vi "Digitizer_Mode_Read.vi"(8 "error in":errorcluster, 11 "Channel Parameters In":T1) -> (0 "error out":errorcluster, 1 "Waveforms Out":T2(array[cluster]), 2 "Ch1_Plot":dbl[](array[numeric]), 3 "dup Channel Parameters Out":T1)   [LabVIEW 2010]
uses:
  Typedef-Channel Parameters.ctl
  <instrlib>/niScope/Acquire/Fetch/niScope Multi Fetch Cluster.vi
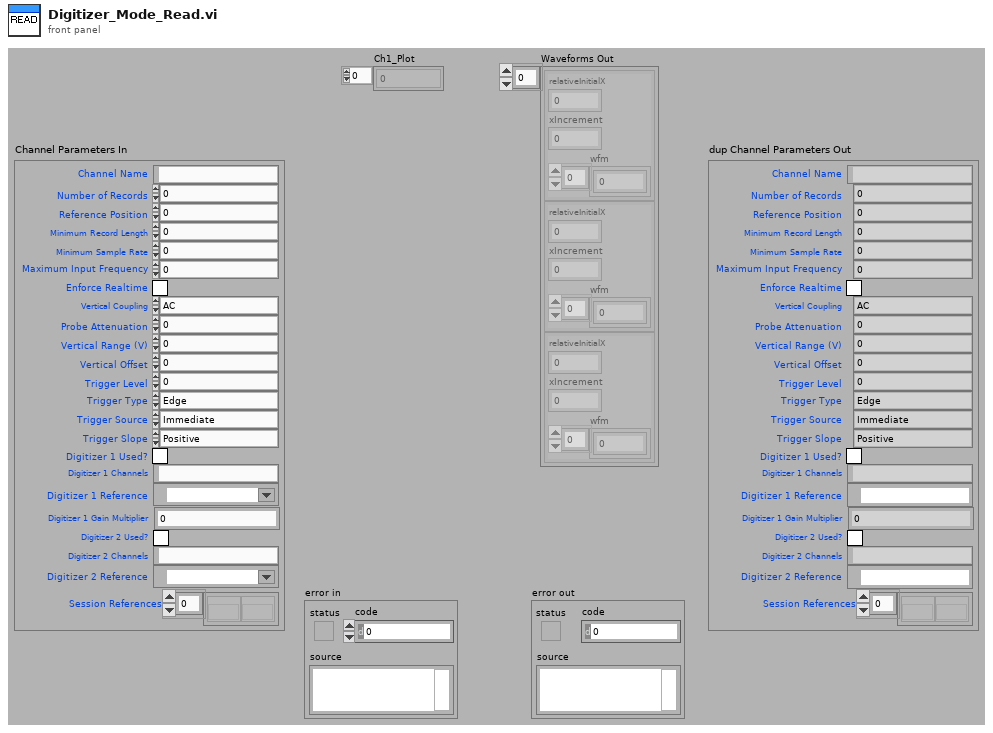
[diagram p1: front panel]
types:
  T1 = typedef "Typedef-Channel Parameters.ctl" = cluster{"Channel Name":string, "Number of Records":i32, "Reference Position":dbl, "Minimum Record Length":i32, "Minimum Sample Rate":dbl, "Maximum Input Frequency":dbl, "Enforce Realtime":bool, "Vertical Coupling":enum16{"AC", "DC", "Ground"}, "Probe Attenuation":dbl, "Vertical Range (V)":dbl, "Vertical Offset":dbl, "Trigger Level":dbl, "Trigger Type":enum16{"Edge", "Digital", "Immediate"}, "Trigger Source":enum16{"Immediate", "Channel 0", "Channel 1", "Channel 2", "Channel 3", "Channel 4", "Channel 5", "Channel 6", "Channel 7", "Extermal TRIG", "Software Trigger", "RTSI 0", "RTSI 1", "RTSI 2", "RTSI 3", "RTSI 4", "RTSI 5", "RTSI 6", "PF 0", "PF 1", "PF 2", "PXI Star Trigger"}, "Trigger Slope":enum16{"Positive", "Negative"}, "Digitizer 1 Used?":bool, "Digitizer 1 Channels":string, "Digitizer 1 Reference":refnum<k15>, "Digitizer 1 Gain Multiplier":dbl, "Digitizer 2 Used?":bool, "Digitizer 2 Channels":string, "Digitizer 2 Reference":refnum<k15>, "Session References":refnum<k20>[]}
  T2 = cluster{"relativeInitialX":dbl, "xIncrement":dbl, "wfm":dbl[]}[]
  T3 = cluster{"relativeInitialX":dbl, "xIncrement":dbl, "wfm":dbl[]}
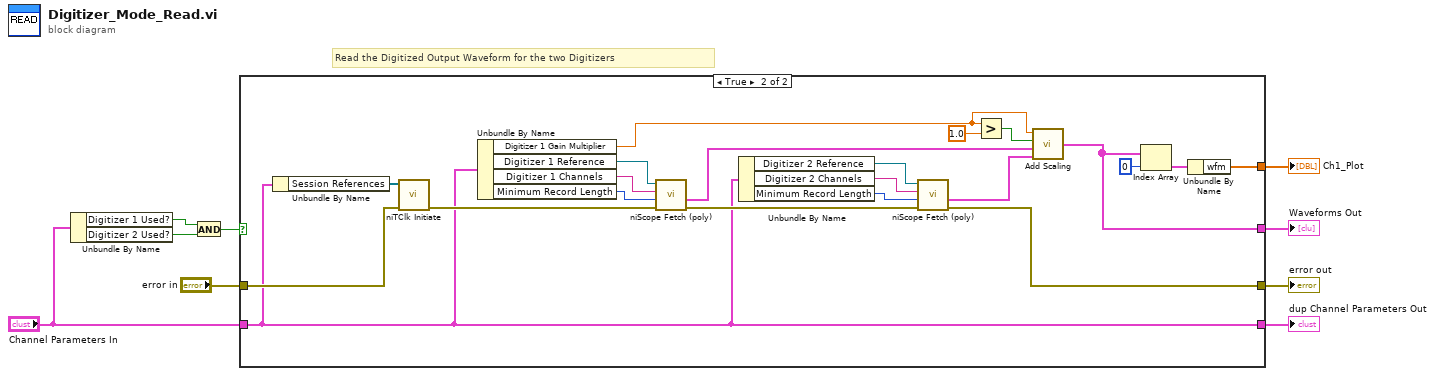
[diagram p0: block diagram]
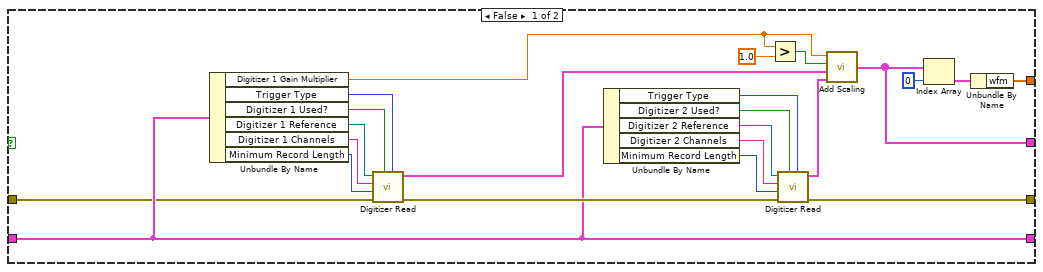
[diagram p2: hidden frame]
diagram:
  # "Read the Digitized Output Waveform for the two Digitizers"
  n1 = Unbundle By Name("Channel Parameters In") -> ("Digitizer 1 Used?"=w6:bool, "Digitizer 2 Used?"=w5:bool)
  n2 = And(x=w6, y=w5) -> (x .and. y?=w3:bool)
  n3 = case shown="True" w3 {
    tunnel: [w30 w35] -> w9
    tunnel: [w27 w39] -> w8
    tunnel: [w16 w36] -> w7
    tunnel: "Channel Parameters In" -> [w11 w33]
    tunnel: [w11 w33] -> w2
    tunnel: "error in" -> [w10 w53]
    frame False {
      n4 = Unbundle By Name(w11) -> ("Digitizer 1 Gain Multiplier"=w32:dbl, "Trigger Type"=w17:enum16{"Edge", "Digital", "Immediate"}, "Digitizer 1 Used?"=w18:bool, "Digitizer 1 Reference"=w13:refnum<k15>, "Digitizer 1 Channels"=w19:string, "Minimum Record Length"=w20:i32)
      n5 = call "Digitizer Read.vi"("Trigger Type"=w17, "Dig Used"=w18, "error in"=w10, "Min Record Length"=w20, "Dig Channels"=w19, "Dig Ref"=w13) -> ("error out"=w21:errorcluster, "waveform out"=w28:T2)  [unwired: 4 in]
      n6 = Unbundle By Name(w11) -> ("Trigger Type"=w22:enum16{"Edge", "Digital", "Immediate"}, "Digitizer 2 Used?"=w23:bool, "Digitizer 2 Reference"=w24:refnum<k15>, "Digitizer 2 Channels"=w25:string, "Minimum Record Length"=w26:i32)
      n7 = Greater?(x=w32, y=1.0) -> (0:w31:bool)
      n8 = call "Digitizer Read.vi"("Trigger Type"=w22, "Dig Used"=w23, "error in"=w21, "Min Record Length"=w26, "Dig Channels"=w25, "Dig Ref"=w24) -> ("error out"=w27:errorcluster, "waveform out"=w29:T2)  [unwired: 4 in]
      n9 = call "Add Scaling.vi"("Digitizer 2 Waveforms"=w29, "Digitizer 1 Waveforms"=w28, "Add Tegam Scaling?"=w31, "Digitizer 1 Gain Multiplier"=w32) -> ("Waveforms Out"=w30:T2)
      n10 = Index Array(array=w30, index=0) -> (element=w15:T3)
      n11 = Unbundle By Name(w15) -> ("wfm"=w16:dbl[])
    }
    frame True {
      n12 = Unbundle By Name(w33) -> ("Session References"=w34:refnum<k20>[])
      n13 = call <instrlib>:"niTClk Initiate.vi"("error in (no error)"=w53, "sessions"=w34) -> ("error out"=w52:errorcluster)  [unwired: 8 in, 1 out]
      n14 = Unbundle By Name(w33) -> ("Digitizer 1 Gain Multiplier"=w40:dbl, "Digitizer 1 Reference"=w50:refnum<k15>, "Digitizer 1 Channels"=w51:string, "Minimum Record Length"=w49:i32)
      n15 = call-poly <instrlib>:"niScope Fetch (poly).vi"("error in"=w52, "numSamples"=w49, "channels"=w51, "instrument handle"=w50) -> ("error out"=w45:errorcluster, "waveform"=w42:T2)  [unwired: 4 in, 2 out]
      n16 = Unbundle By Name(w33) -> ("Digitizer 2 Reference"=w48:refnum<k15>, "Digitizer 2 Channels"=w47:string, "Minimum Record Length"=w46:i32)
      n17 = call-poly <instrlib>:"niScope Fetch (poly).vi"("error in"=w45, "numSamples"=w46, "channels"=w47, "instrument handle"=w48) -> ("error out"=w39:errorcluster, "waveform"=w41:T2)  [unwired: 4 in, 2 out]
      n18 = Greater?(x=w40, y=1.0) -> (0:w44:bool)
      n19 = call "Add Scaling.vi"("Digitizer 2 Waveforms"=w41, "Digitizer 1 Waveforms"=w42, "Add Tegam Scaling?"=w44, "Digitizer 1 Gain Multiplier"=w40) -> ("Waveforms Out"=w35:T2)
      n20 = Index Array(array=w35, index=0) -> (element=w38:T3)
      n21 = Unbundle By Name(w38) -> ("wfm"=w36:dbl[])
    }
  }
  "Ch1_Plot" <- w7
  "Waveforms Out" <- w9
  "error out" <- w8
  "dup Channel Parameters Out" <- w2
